vi "initialise.vi"(8 "error in (no error)":errorcluster, 11 "GenericPlugin in":refnum<class "FPGAWrapperDL090211Galvo_grabber.lvclass">) -> (0 "error out":errorcluster, 3 "GenericPlugin out":refnum<class "FPGAWrapperDL090211Galvo_grabber.lvclass">)   [LabVIEW 2010, in "FPGAWrapperDL090211Galvo_grabber.lvclass"]
doc: "The dynamic dispatch-version of this VI initalises the plug-in object by allocating and initalising any dynamic resources need."
uses:
  FPGAWrapperDL090211Galvo_grabber.lvclass
  GenericFPGAWrapper/GenericFPGAWrapper/GenericFPGAWrapper.lvclass
  FPGAWrapperDL090211Galvo_grabber.lvclass/FPGAWrapperDL090211Galvo_grabber.ctl
  type definitions/command_enum.ctl
  class_data.vi
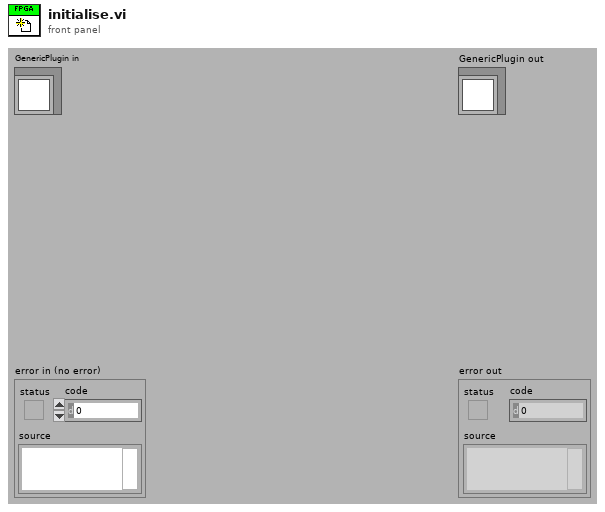
[diagram p1: front panel]
types:
  T1 = typedef "command_enum.ctl" = enum16{"NULL", "update", "start", "stop", "reset", "shut-down"}
  T2 = typedef "config_data_cluster.ctl" = cluster{"bit file":string, "hifo box version":i32, "ADC clock phase":i32}
  T3 = typedef "settings_cluster.ctl" = cluster{"number of pixels":i32, "iterations per pixel":i32, "maximum bit-depth":i32, "pixel values cluster":T4, "triggered?":bool, "triggered flag valid?":bool, "gates":T5[]}
  T4 = typedef "channels_cluster.ctl" = cluster{"channel 0":u32, "channel 1":u32, "channel 2":u32, "channel 3":u32}
  T5 = typedef "gate_cluster.ctl" = cluster{"index":i32, "parameters":T6}
  T6 = typedef "gate_parameters_cluster.ctl" = cluster{"offset":i64, "pulsing":i64, "not pulsing":i64, "cycles per pulse":i64, "repetitions":i64}
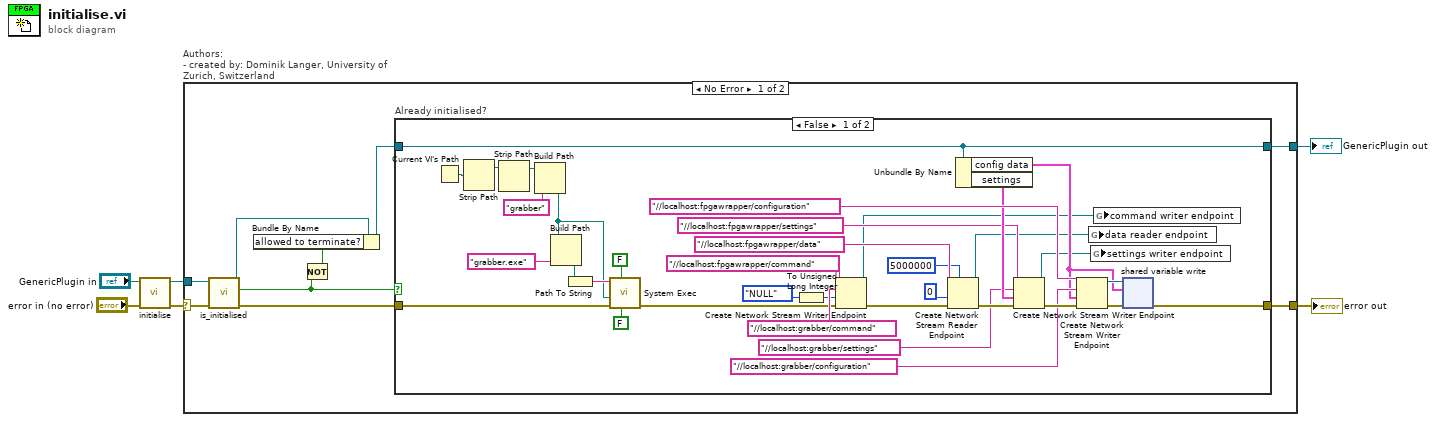
[diagram p0: block diagram]
diagram:
  n1 = call-parent "initialise.vi"("error in (no error)"="error in (no error)", "GenericPlugin in"="GenericPlugin in") -> ("error out"=w4:errorcluster, "GenericPlugin out"=w3:refnum<class "FPGAWrapperDL090211Galvo_grabber.lvclass">)  [unwired: 8 in]
  n2 = case "Authors: \n- created by: Dominik Langer, University of Zurich, Switzerland" shown="No Error" w4 {
    selector: w4 -> [w14 w53]
    tunnel: w3 -> [w13 w54]
    tunnel: [w15 w53] -> w2
    tunnel: [w11 w54] -> w1
    frame No Error {
      n3 = call-dynamic "is_initialised.vi"("error in (no error)"=w14, "FPGAWrapperDL120115Galvo in"=w13) -> ("error out"=w12:errorcluster, "is initialised?"=w8:bool, "FPGAWrapperDL120115Galvo out"=w10:refnum<class "FPGAWrapperDL090211Galvo_grabber.lvclass">)  [unwired: 7 in]
      n4 = Not(x=w8) -> (.not. x?=w7:bool)
      n5 = Bundle By Name(cluster=w10, "allowed to terminate?"=w7) -> (w9:refnum<class "FPGAWrapperDL090211Galvo_grabber.lvclass">)
      n6 = case "Already initialised?" shown="False" w8 {
        tunnel: w12 -> [w19 w51]
        tunnel: [w18 w52] -> w11
        tunnel: w9 -> [w18 w52]
        tunnel: [w39 w51] -> w15
        frame False {
          n7 = Current VI's Path() -> (path=w29:path)
          n8 = Strip Path(path=w29) -> (stripped path=w30:path)  [unwired: 1 out]
          n9 = Strip Path(path=w30) -> (stripped path=w32:path)  [unwired: 1 out]
          n10 = Build Path(base path=w32, name or relative path="grabber") -> (appended path=w20:path)
          n11 = Build Path(base path=w20, name or relative path="grabber.exe" ("command line")) -> (appended path=w26:path)
          n12 = Path To String(path=w26) -> (string=w27:string)
          n13 = call <vilib>:"System Exec.vi"("run minimized? (F)"=FALSE, "wait until completion? (T)"=FALSE, "error in (no error)"=w19, "working directory"=w20, "command line"=w27) -> ("error out"=w28:errorcluster)  [unwired: 3 in, 3 out]
          n14 = To Unsigned Long Integer(number=command_enum."NULL" ("command")) -> (unsigned 32bit integer=w48:u32)
          n15 = Create Network Stream Writer Endpoint(8:w28, 9:w48, 10:"//localhost:grabber/command" ("writer name"), 11:"//localhost:fpgawrapper/command" ("writer name")) -> (0:w46:errorcluster, 3:w23:refnum<k21>)  [unwired: 2 in]
          n16 = Create Network Stream Reader Endpoint(7:5000000 ("reader buffer size"), 8:w46, 9:u64 0, 11:"//localhost:fpgawrapper/data" ("reader url")) -> (0:w41:errorcluster, 3:w22:refnum<k21>)  [unwired: 2 in]
          n17 = Unbundle By Name(w18) -> ("config data"=w34:T2, "settings"=w42:T3)
          n18 = Create Network Stream Writer Endpoint(8:w41, 9:w42, 10:"//localhost:grabber/settings" ("writer name"), 11:"//localhost:fpgawrapper/settings" ("writer name")) -> (0:w40:errorcluster, 3:w21:refnum<k21>)  [unwired: 2 in]
          n19 = Create Network Stream Writer Endpoint(8:w40, 9:w34, 10:"//localhost:grabber/configuration" ("reader url"), 11:"//localhost:fpgawrapper/configuration" ("writer name")) -> (0:w43:errorcluster, 3:w44:refnum<k21>)  [unwired: 2 in]
          n20 = global write "class_data.vi" "data reader endpoint"(w22) -> ()
          n21 = global write "class_data.vi" "settings writer endpoint"(w21) -> ()
          n22 = global write "class_data.vi" "command writer endpoint"(w23) -> ()
          n23 = shared-variable-write(w44, w43, w34) -> (w39:errorcluster)  [unwired: 1 in, 2 out]
        }
        frame True {
        }
      }
    }
    frame Error {
    }
  }
  "error out" <- w2
  "GenericPlugin out" <- w1
